vi "aoc-2025-d03-2.vi"() -> ()   [LabVIEW 2020]
panel:
  out "numbers":i64[](array[numeric])
  out "sum":i64
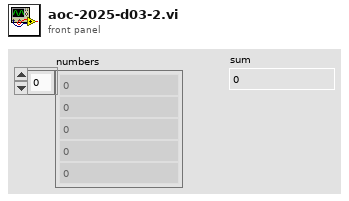
[diagram p1: front panel]
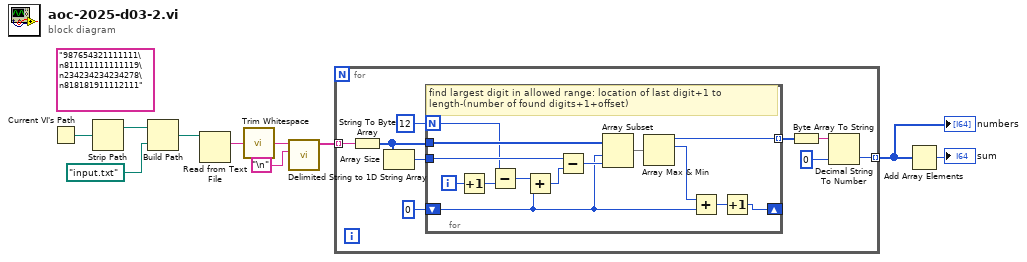
[diagram p0: block diagram]
diagram:
  (unwired) "987654321111111\n811111111111119\n234234234234278\n818181911112111"
  n1 = Current VI's Path() -> (path=w7:path)
  n2 = Strip Path(path=w7) -> (stripped path=w6:path)  [unwired: 1 out]
  n3 = Build Path(base path=w6, name or relative path=path "input.txt") -> (appended path=w4:path)
  n4 = Read from Text File(file (use dialog)=w4) -> (text=w1:string)  [unwired: 3 in, 3 out]
  n5 = call <vilib>:"Trim Whitespace.vi"("string"=w1) -> ("trimmed string"=w3:string)  [unwired: 1 in]
  n6 = call <vilib>:"Delimited String to 1D String Array.vi"("delimiter"="\n", "delimited string"=w3) -> ("string array"=w2:string[])  [unwired: 9 in]
  n7 = for {
    tunnel: w2 -> [w19] mode=indexing
    tunnel: [w17] -> w8 mode=indexing
    n8 = String To Byte Array(string=w19) -> (unsigned byte array=w11:u8[])
    n9 = Array Size(array=w11) -> (size(s)=w15:i32)
    n10 = for {
      N: 12 -> [w31]
      tunnel: w11 -> [w33]
      tunnel: w15 -> [w32]
      tunnel: [w30] -> w14 mode=indexing
      shift-right: [w27] -> _
      shift-left: 0 -> [w21]
      i -> [w25]
      # "find largest digit in allowed range: location of last digit+1 to length-(number of found digits+1+offset)"
      n11 = Increment(x=w25) -> (x+1=w24:i32)
      n12 = Subtract(x=w31, y=w24) -> (x-y=w23:i32)
      n13 = Add(x=w23, y=w21) -> (x+y=w20:i32)
      n14 = Subtract(x=w32, y=w20) -> (x-y=w22:i32)
      n15 = Array Subset(array=w33, index=w21, length=w22) -> (w26:u8[])
      n16 = Array Max & Min(array=w26) -> (max value=w30:u8, max index (indices)=w29:i32)  [unwired: 2 out]
      n17 = Add(x=w29, y=w21) -> (x+y=w28:i32)
      n18 = Increment(x=w28) -> (x+1=w27:i32)
    }
    n19 = Byte Array To String(unsigned byte array=w14) -> (string=w18:string)
    n20 = Decimal String To Number(string=w18, default (0L)=i64 0 ("default (0 I32)")) -> (number=w17:i64)  [unwired: 1 in, 1 out]
  }
  "numbers" <- w8
  n21 = Add Array Elements(numeric array=w8) -> (sum=→"sum":i64)
